vi "motor4 position control.vi"(6 "error in (no error)":errorcluster, 8 "Goal Speed (RPM)":dbl, 9 "Goal Position (180 deg)":dbl=180.0, 10 "Motor ID (0)":u8, 11 "VISA resource name":refnum<visa-resource-name>) -> (3 "VISA resource name out":refnum<visa-resource-name>, 4 "error out":errorcluster)   [LabVIEW 2016]
uses:
  <instrlib>/Dynamixel Motor/Dynamixel Motor.lvlib
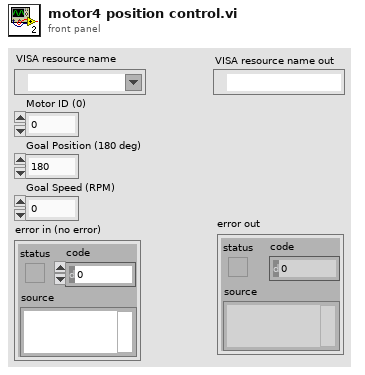
[diagram p1: front panel]
types:
  T1 = enum16{"big-endian, network order", "native, host order", "little-endian"}
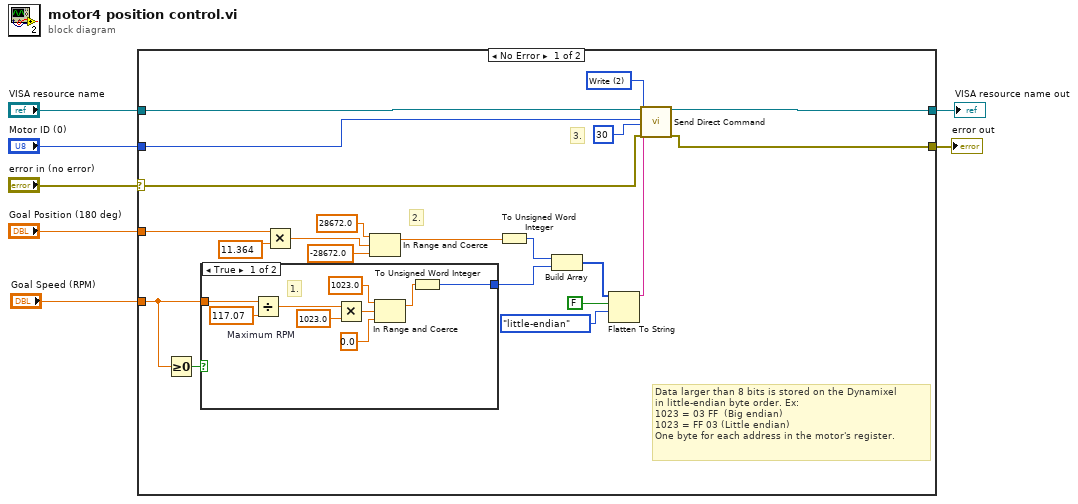
[diagram p0: block diagram]
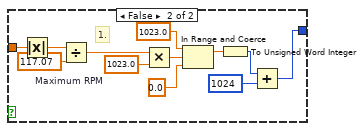
[diagram p2: hidden frame]
diagram:
  n1 = case shown="No Error" "error in (no error)" {
    selector: "error in (no error)" -> [w14 w51]
    tunnel: "VISA resource name" -> [w27 w50]
    tunnel: [w26 w50] -> w6
    tunnel: [w25 w51] -> w5
    tunnel: "Motor ID (0)" -> [w24 _]
    tunnel: "Goal Position (180 deg)" -> [w21 _]
    tunnel: "Goal Speed (RPM)" -> [w8 _]
    frame No Error {
      w28 = u16 2 items=["Ping", "Read", "Write", "Registered Write", "Action", "Reset", "Sync Write"] ("Select Action")
      # "3."
      # "2."
      # "Data larger than 8 bits is stored on the Dynamixel \nin little-endian byte order. Ex:\n1023 = 03 FF  (Big endian)\n1023 = FF 03 (Little endian)\nOne byte for each address in the motor's register."
      n2 = Greater Or Equal To 0?(x=w8) -> (x >= 0?=w9:bool)
      n3 = case shown="True" w9 {
        tunnel: w8 -> [w34 w46]
        tunnel: [w30 w39] -> w17
        frame True {
          w31 = 117.07  # Maximum RPM
          # "1."
          n4 = Divide(x=w34, y=w31) -> (x/y=w33:dbl)
          n5 = Multiply(x=w33, y=1023.0 ("upper limit")) -> (x*y=w37:dbl)
          n6 = In Range and Coerce(upper limit=1023.0, x=w37, lower limit=0.0) -> (coerced(x)=w29:dbl)  [unwired: 1 out]
          n7 = To Unsigned Word Integer(number=w29) -> (unsigned 16bit integer=w30:u16)
        }
        frame False {
          w43 = 117.07  # Maximum RPM
          # "1."
          n8 = Absolute Value(x=w46) -> (abs(x)=w41:dbl)
          n9 = Divide(x=w41, y=w43) -> (x/y=w45:dbl)
          n10 = Multiply(x=w45, y=1023.0 ("upper limit")) -> (x*y=w49:dbl)
          n11 = In Range and Coerce(upper limit=1023.0, x=w49, lower limit=0.0) -> (coerced(x)=w42:dbl)  [unwired: 1 out]
          n12 = To Unsigned Word Integer(number=w42) -> (unsigned 16bit integer=w40:u16)
          n13 = Add(x=w40, y=u16 1024) -> (x+y=w39:u16)
        }
      }
      n14 = Multiply(x=w21, y=11.364) -> (x*y=w11:dbl)
      n15 = In Range and Coerce(upper limit=28672.0, x=w11, lower limit=-28672.0) -> (coerced(x)=w10:dbl)  [unwired: 1 out]
      n16 = To Unsigned Word Integer(number=w10) -> (unsigned 16bit integer=w18:u16)
      n17 = Build Array(w18, w17) -> (w16:u16[])
      n18 = Flatten To String(anything=w16, prepend array or string size? (T)=FALSE, byte order (0:big-endian, network order)=T1."little-endian") -> (data string=w15:string)  [unwired: 1 in, 2 out]
      n19 = call <instrlib>:"Send Direct Command.vi"("VISA resource name"=w27, "Select Action"=w28, "Motor ID (0)"=w24, "Address"=u8 30, "Parameters"=w15, "Error in (no error)"=w14) -> ("VISA resource name out"=w26:refnum<visa-resource-name>, "Error out"=w25:errorcluster)  [unwired: 11 in, 1 out]
    }
    frame Error {
    }
  }
  "VISA resource name out" <- w6
  "error out" <- w5
